vi "Close_Session.vi"(1 "error in (no error)":errorcluster, 2 "Read Session":refnum<k21>, 3 "Write Session":refnum<k21>) -> (0 "error out":errorcluster)   [LabVIEW 2023]
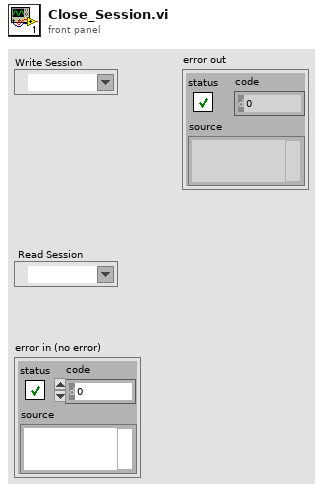
[diagram p1: front panel]
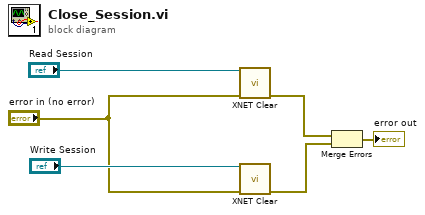
[diagram p0: block diagram]
diagram:
  n1 = call <vilib>:"XNET Clear.vi"("session in"="Read Session", "error in (no error)"="error in (no error)") -> ("error out"=w3:errorcluster)  [unwired: 13 in]
  n2 = call <vilib>:"XNET Clear.vi"("session in"="Write Session", "error in (no error)"="error in (no error)") -> ("error out"=w2:errorcluster)  [unwired: 13 in]
  n3 = Merge Errors(w3, w2) -> (→"error out":errorcluster)
